vi "CTTC_AiP_Channel_Mapping.vi"(7 "AiP":u16(ring)=1 items=["AiP_1"=1, "AiP_2"=2, "AiP_3"=3, "AiP_4"=4]) -> (1 "Pol_V":i32[](array[numeric]), 2 "Pol_H":i32[](array[numeric]), 3 "Ch_Index":i32[](array[numeric]))   [LabVIEW 2023]
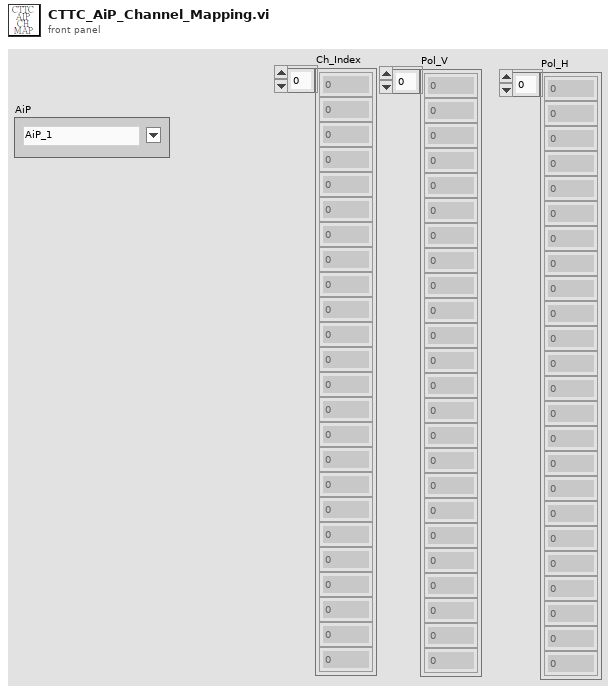
[diagram p1: front panel]
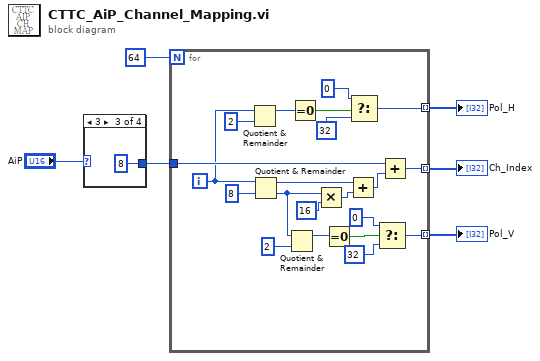
[diagram p0: block diagram]
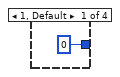
[diagram p2: hidden frame]
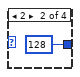
[diagram p3: hidden frame]
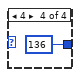
[diagram p4: hidden frame]
diagram:
  n1 = case shown="3" "AiP" {
    tunnel: [0 ("y") 128 ("y") 8 ("y") 136 ("y")] -> w3
    frame 1, Default {
    }
    frame 2 {
    }
    frame 3 {
    }
    frame 4 {
    }
  }
  n2 = for {
    N: 64 -> [_]
    tunnel: [w26] -> w5 mode=indexing
    tunnel: w3 -> [w27]
    tunnel: [w21] -> w2 mode=indexing
    tunnel: [w11] -> w1 mode=indexing
    i -> [w20]
    n3 = Quotient & Remainder(x=w20, y=2) -> (x-y*floor(x/y)=w18:i32)  [unwired: 1 out]
    n4 = Quotient & Remainder(x=w20, y=8) -> (x-y*floor(x/y)=w25:i32, floor(x/y)=w16:i32)
    n5 = Quotient & Remainder(x=w16, y=2) -> (x-y*floor(x/y)=w13:i32)  [unwired: 1 out]
    n6 = Equal To 0?(x=w18) -> (x = 0?=w24:bool)
    n7 = Multiply(x=w16, y=16) -> (x*y=w29:i32)
    n8 = Equal To 0?(x=w13) -> (x = 0?=w12:bool)
    n9 = Add(x=w25, y=w29) -> (x+y=w28:i32)
    n10 = Select(t=0 ("Phase"), s=w24, f=32 ("Phase")) -> (s? t:f=w21:i32)
    n11 = Select(t=0 ("Phase"), s=w12, f=32 ("Phase")) -> (s? t:f=w11:i32)
    n12 = Add(x=w27, y=w28) -> (x+y=w26:i32)
  }
  "Ch_Index" <- w5
  "Pol_V" <- w1
  "Pol_H" <- w2
